vi "Splash Screen.vi"() -> ()   [LabVIEW 2017, in "Package Building Launcher.lvlib"]
doc: "This is the top-level VI of this application. When it runs, it behaves like the splash screen many applications use to keep the user occupied while the application loads into memory. This application is quite small, so there is little overhead, which would make the splash screen just flash for a moment. Because that flash is distracting, there is a three-second delay inserted into this VI so that it stays up for a little bit. \n\nThis VI uses a delay-loaded subVI call to load the rest of the application. This trick ensures that the splash screen can load instantly regardless of how large the rest of the VI hierarchy gets, and the loading of the rest of the VIs becomes one step in the load process."
uses:
  Package Building Launcher.lvlib
  Pacjage Building/Pacjage Building/Load App.vi
  Pacjage Building/Pacjage Building/Package Building.lvclass
panel:
  out "Waiting Lights":T1
  out "Application Name":string
  out "Current Action":string caption="Current action:"
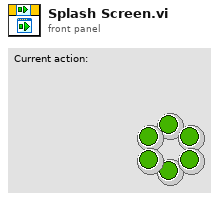
[diagram p1: front panel]
types:
  T1 = cluster{"wait 1":bool, "wait 2":bool, "wait 3":bool, "wait 4":bool, "wait 5":bool, "wait 6":bool}
  T2 = cluster{"[0]":bool, "[1]":bool, "[2]":bool, "[3]":bool, "[4]":bool, "[5]":bool}
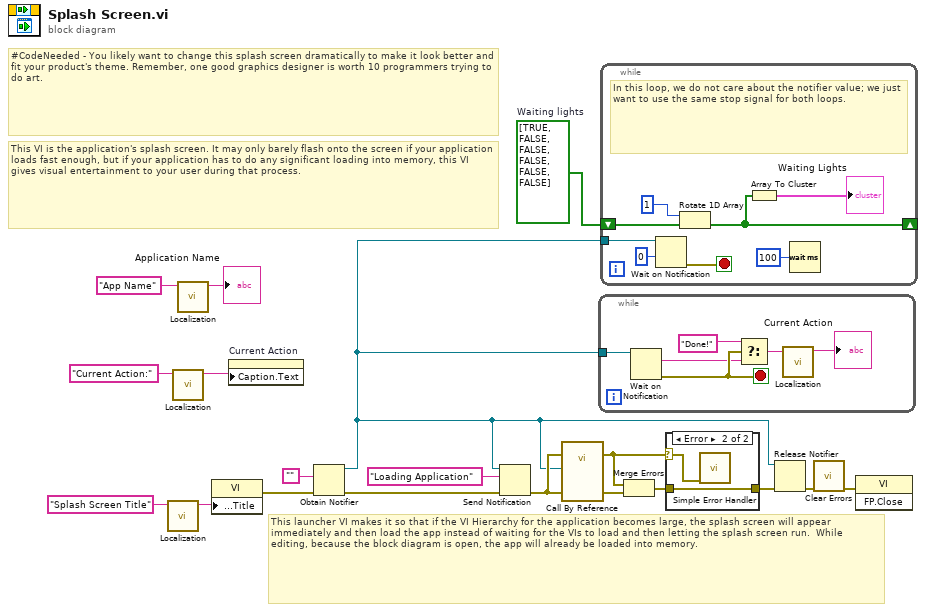
[diagram p0: block diagram]
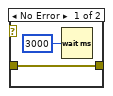
[diagram p2: hidden frame]
diagram:
  w8 = bool[] [TRUE, FALSE, FALSE, FALSE, FALSE, FALSE]  # Waiting lights
  # "#CodeNeeded - You likely want to change this splash screen dramatically to make it look better and fit your product's theme. Remember, one good graphics designer is worth 10 programmers trying to do art."
  # "This VI is the application's splash screen. It may only barely flash onto the screen if your application loads fast enough, but if your application has to do any significant loading into memory, this VI gives visual entertainment to your user during that process."
  # "This launcher VI makes it so that if the VI Hierarchy for the application becomes large, the splash screen will appear immediately and then load the app instead of waiting for the VIs to load and then letting the splash screen run.  While editing, because the block diagram is open, the app will already be loaded into memory."
  n1 = call "Localization.vi"("Unlocalized"="Splash Screen Title" ("Window Title")) -> ("Localized"=w19:string)  [unwired: 10 in]
  n2 = call "Localization.vi"("Unlocalized"="Current Action:" ("Window Title")) -> ("Localized"=w4:string)  [unwired: 10 in]
  n3 = call "Localization.vi"("Unlocalized"="App Name") -> ("Localized"=→"Application Name":string)  [unwired: 10 in]
  n4 = property class="VI"("Front Panel.Title"=w19) -> (error out=w17:errorcluster)  [unwired: 2 in, 1 out]
  n5 = property on="Current Action" class="Str"("Caption.Text"=w4) -> ()  [unwired: 2 in, 2 out]
  n6 = Obtain Notifier(notification data type="", error in (no error)=w17) -> (notifier out=w12:refnum<notifier>, error out=w6:errorcluster)  [unwired: 2 in, 1 out]
  n7 = Send Notification(notification="Loading Application", notifier=w12, error in (no error)=w6) -> (error out=w13:errorcluster)  [unwired: 1 out]
  n8 = call-by-ref "?"(error in=w13, 8:"error in (no error)"=w13, "Status Notifier"=w12) -> (error out=w1:errorcluster, 0:"error out"=w16:errorcluster)  [unwired: 10 in, 1 out]
  n9 = while {
    tunnel: w12 -> [w24]
    stop <- w23 stop-if-true
    n10 = Wait on Notification(notifier=w24) -> (notification=w21:string, error out=w23:errorcluster)  [unwired: 3 in, 2 out]
    n11 = Select(t="Done!" ("notification"), s=w23, f=w21) -> (s? t:f=w20:string)
    n12 = call "Localization.vi"("Unlocalized"=w20) -> ("Localized"=→"Current Action":string)  [unwired: 10 in]
  }
  n13 = while {
    shift-right: [w27] -> _
    shift-left: w8 -> [w29]
    tunnel: w12 -> [w31]
    stop <- w33 stop-if-true
    # "In this loop, we do not care about the notifier value; we just want to use the same stop signal for both loops."
    n14 = Wait on Notification(notifier=w31, timeout in ms (-1)=0) -> (error out=w33:errorcluster)  [unwired: 2 in, 3 out]
    n15 = Rotate 1D Array(1:w29, 2:1 ("n")) -> (0:w27:bool[])
    n16 = Array To Cluster(array=w27) -> (cluster=→"Waiting Lights":T2)
    n17 = Wait (ms)(milliseconds to wait=u32 100) -> ()  [unwired: 1 out]
  }
  n18 = Merge Errors(w1, w16) -> (w2:errorcluster)
  n19 = case shown="Error" w1 {
    tunnel: [w35 w36] -> w3
    tunnel: w2 -> [w35 w36]
    selector: w1 -> [_ w37]
    frame No Error {
      n20 = Wait (ms)(milliseconds to wait=u32 3000) -> ()  [unwired: 1 out]
    }
    frame Error {
      n21 = call <vilib>:"Simple Error Handler.vi"("error in (no error)"=w37) -> ()  [unwired: 4 in, 5 out]
    }
  }
  n22 = Release Notifier(notifier=w12, error in (no error)=w3) -> (error out=w15:errorcluster)  [unwired: 1 in, 2 out]
  n23 = call <vilib>:"Clear Errors.vi"("error in (no error)"=w15) -> ("error out"=w7:errorcluster)  [unwired: 5 in, 1 out]
  n24 = invoke class="VI" method="FP.Close"(error in=w7) -> ()  [unwired: 2 in, 3 out]
